vi "ConfigureEcMotorTypeEx.vi"(4 "error in (no error)":errorcluster, 5 "motor type":u16(ring)=11 items=["EC motor (sinus commutated)"=10, "EC motor (block commutated)"=11], 6 "EC motor parameter ex":T1, 7 "axis in":cluster{"keyHandle":u32, "nodeId":u16}={"keyHandle"=0, "nodeId"=1}) -> (0 "error out":errorcluster, 3 "axis out":cluster{"keyHandle":u32, "nodeId":u16}={"keyHandle"=0, "nodeId"=1})   [LabVIEW 2017, in "maxonEPOS.lvlib"]
doc: "<B>ConfigureEcMotorType</B> writes the value for DC motor type to the device. Parameters for the EC motor type can be set."
uses:
  Examples/maxonEPOS.lvlib
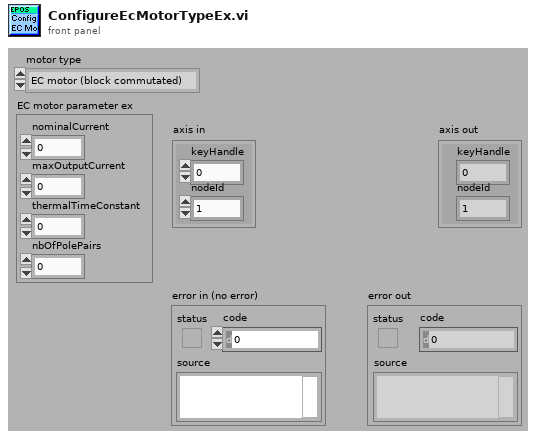
[diagram p1: front panel]
types:
  T1 = cluster{"nominalCurrent":u32, "maxOutputCurrent":u32, "thermalTimeConstant":u16, "nbOfPolePairs":u8}
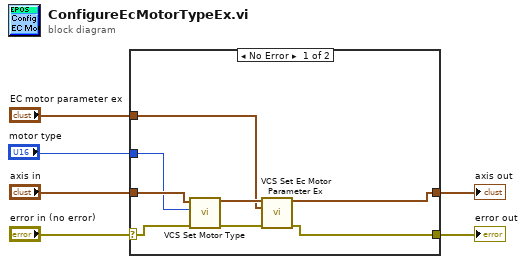
[diagram p0: block diagram]
diagram:
  n1 = case shown="No Error" "error in (no error)" {
    selector: "error in (no error)" -> [w14 w16]
    tunnel: [w8 w16] -> w5
    tunnel: [w7 w15] -> w4
    tunnel: "axis in" -> [w11 w15]
    tunnel: "motor type" -> [w10 _]
    tunnel: "EC motor parameter ex" -> [w9 _]
    frame No Error {
      n2 = call "VCS Set Motor Type.vi"("error in (no error)"=w14, "motor type"=w10, "axis in"=w11) -> ("error out"=w13:errorcluster, "axis out"=w12:cluster{"keyHandle":u32, "nodeId":u16})  [unwired: 7 in]
      n3 = call "VCS Set Ec Motor Parameter Ex.vi"("axis in"=w12, "EC motor parameter ex"=w9, "error in (no error)"=w13) -> ("axis out"=w7:cluster{"keyHandle":u32, "nodeId":u16}, "error out"=w8:errorcluster)  [unwired: 11 in]
    }
    frame Error {
    }
  }
  "error out" <- w5
  "axis out" <- w4
